vi "Static test.vi"(0 "SceneObject in":refnum<vi>, 3 "data (can be any type)":string, 5 "Child 3":refnum<vi>, 7 "Child 2":refnum<vi>, 9 "Child":refnum<vi>) -> (4 "SceneNode out":refnum<vi>(3d-picture), 6 "number":dbl, 8 "number 2":dbl, 10 "number 3":dbl, 14 "number 5":dbl, 15 "number 4":dbl)   [LabVIEW 2020]
uses:
  <vilib>/picture/3D Picture Control/NI_3D Picture Control.lvlib
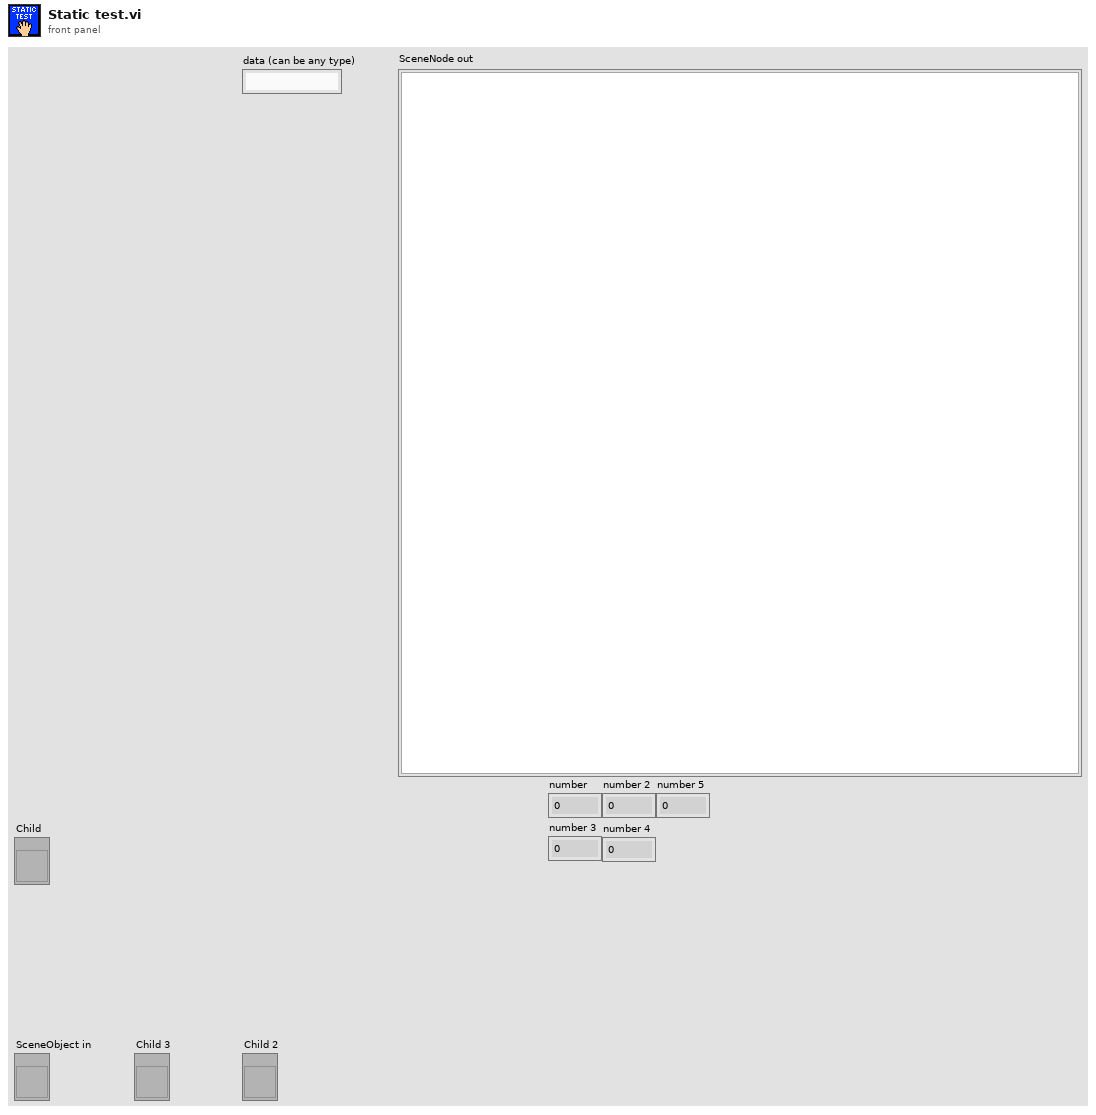
[diagram p1: front panel]
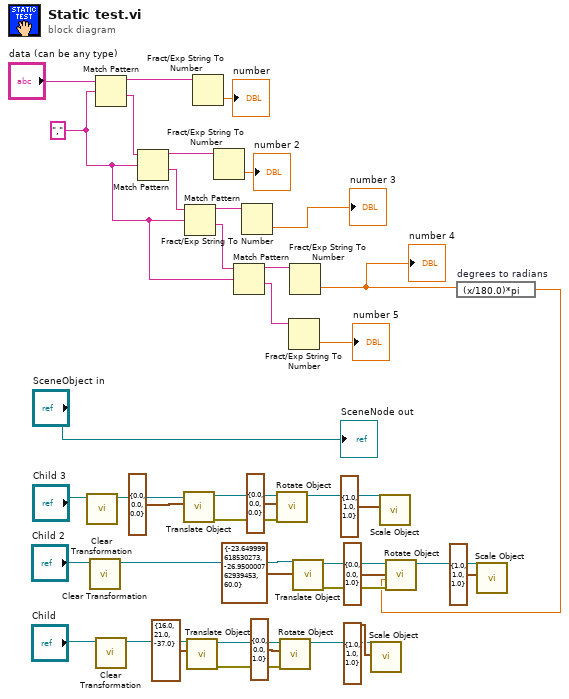
[diagram p0: block diagram]
diagram:
  w2 = ","
  n1 = call <vilib>:"Clear Transformation.vi"("Object Refnum In"="Child 3") -> ("Object Refnum Out"=w20:refnum<vi>)  [unwired: 9 in, 1 out]
  n2 = call <vilib>:"Clear Transformation.vi"("Object Refnum In"="Child 2") -> ("Object Refnum Out"=w7:refnum<vi>)  [unwired: 9 in, 1 out]
  n3 = Match Pattern(string="data (can be any type)", regular expression=w2) -> (before substring=w37:string, after substring=w38:string)  [unwired: 1 in, 2 out]
  n4 = call <vilib>:"Clear Transformation.vi"("Object Refnum In"="Child") -> ("Object Refnum Out"=w30:refnum<vi>)  [unwired: 9 in, 1 out]
  n5 = Match Pattern(string=w38, regular expression=w2) -> (before substring=w39:string, after substring=w11:string)  [unwired: 1 in, 2 out]
  n6 = call <vilib>:"Translate Object.vi"("Translation"=cluster{"X":sgl, "Y":sgl, "Z":sgl} {"X"=0.0, "Y"=0.0, "Z"=0.0}, "Scene.Object In"=w20) -> ("error out"=w17:errorcluster, "Scene.Object Out"=w21:refnum<vi>)  [unwired: 8 in]
  n7 = Match Pattern(string=w11, regular expression=w2) -> (before substring=w13:string, after substring=w5:string)  [unwired: 1 in, 2 out]
  n8 = call <vilib>:"Translate Object.vi"("Translation"=cluster{"X":sgl, "Y":sgl, "Z":sgl} {"X"=16.0, "Y"=21.0, "Z"=-37.0} ("Translation 2"), "Scene.Object In"=w30) -> ("error out"=w28:errorcluster, "Scene.Object Out"=w31:refnum<vi>)  [unwired: 8 in]
  n9 = Fract/Exp String To Number(string=w37) -> (number=→"number":dbl)  [unwired: 3 in, 1 out]
  n10 = Fract/Exp String To Number(string=w39) -> (number=→"number 2":dbl)  [unwired: 3 in, 1 out]
  n11 = Match Pattern(string=w5, regular expression=w2) -> (before substring=w4:string, after substring=w3:string)  [unwired: 1 in, 2 out]
  n12 = Fract/Exp String To Number(string=w13) -> (number=→"number 3":dbl)  [unwired: 3 in, 1 out]
  n13 = call <vilib>:"Rotate Object.vi"("error in (no error)"=w17, "Axis"=cluster{"X":sgl, "Y":sgl, "Z":sgl} {"X"=0.0, "Y"=0.0, "Z"=0.0}, "Scene.Object In"=w21) -> ("Scene.Object Out"=w22:refnum<vi>)  [unwired: 7 in, 1 out]
  n14 = call <vilib>:"Rotate Object.vi"("error in (no error)"=w28, "Axis"=cluster{"X":sgl, "Y":sgl, "Z":sgl} {"X"=0.0, "Y"=0.0, "Z"=1.0}, "Scene.Object In"=w31) -> ("Scene.Object Out"=w32:refnum<vi>)  [unwired: 7 in, 1 out]
  n15 = Fract/Exp String To Number(string=w3) -> (number=→"number 5":dbl)  [unwired: 3 in, 1 out]
  n16 = Fract/Exp String To Number(string=w4) -> (number=w12:dbl)  [unwired: 3 in, 1 out]
  "number 4" <- w12
  n17 = call <vilib>:"Translate Object.vi"("Translation"=cluster{"X":sgl, "Y":sgl, "Z":sgl} {"X"=-23.65, "Y"=-26.95, "Z"=60.0}, "Scene.Object In"=w7) -> ("error out"=w24:errorcluster, "Scene.Object Out"=w25:refnum<vi>)  [unwired: 8 in]
  n18 = call <vilib>:"Scale Object.vi"("Scale"=cluster{"X":sgl, "Y":sgl, "Z":sgl} {"X"=1.0, "Y"=1.0, "Z"=1.0}, "Scene.Object In"=w32) -> ()  [unwired: 8 in, 2 out]
  n19 = call <vilib>:"Scale Object.vi"("Scale"=cluster{"X":sgl, "Y":sgl, "Z":sgl} {"X"=1.0, "Y"=1.0, "Z"=1.0}, "Scene.Object In"=w22) -> ()  [unwired: 8 in, 2 out]
  n20 = expression code="(x/180.0)*pi" "degrees to radians"(w12) -> (w6:dbl)
  n21 = call <vilib>:"Rotate Object.vi"("error in (no error)"=w24, "Angle"=w6, "Axis"=cluster{"X":sgl, "Y":sgl, "Z":sgl} {"X"=0.0, "Y"=0.0, "Z"=1.0}, "Scene.Object In"=w25) -> ("Scene.Object Out"=w26:refnum<vi>)  [unwired: 6 in, 1 out]
  n22 = call <vilib>:"Scale Object.vi"("Scale"=cluster{"X":sgl, "Y":sgl, "Z":sgl} {"X"=1.0, "Y"=1.0, "Z"=1.0}, "Scene.Object In"=w26) -> ()  [unwired: 8 in, 2 out]
  "SceneNode out" <- "SceneObject in"
